vi "Test Xiaolei Hu_Several Frame.vi"() -> ()   [LabVIEW 2017]
doc: "Created IvanLis by LabVIEW Portal\nProfile: http://labviewportal.org/memberlist.php?mode=viewprofile&u=987\neMail: IvanLisanov@gMail.com\nTelegram: https://t.me/IvanLis"
uses:
  libonnx_wrapper/libonnx_wrapper.lvlib
  libonnx_wrapper/TypeDef/IO.ctl
  libonnx_wrapper/TypeDef/Introspection.ctl
panel:
  out "change index":i32
  in  "Next Image":bool
  in  "threshold":sgl=0.3 format="%#.6g"
  in  "max Object's":i64=9
  in  "Tab Control":enum32{"Result", "Introspection"}(tab)
  out "detected_boxes":sgl[][](array[numeric])
  out "detected_classes":sgl[](array[numeric])
  out "score":sgl[](array[numeric])
  out "change":bool[](array[boolean])
  out "Introspection Input":T1
  out "Introspection Output":T1
  out "2D Picture":picture
  out "PNG file path":path=path "/home/ivan/LabVIEWData/ONNX/LabVIEW-ONNX_Runtime/image_for_test/1_1_2r_1_1_var10.jpg"
  out "ONNX model path":path=path "/home/ivan/LabVIEWData/ONNX/LabVIEW-ONNX_Runtime/data/coins_detection.onnx"
  out "error out":errorcluster
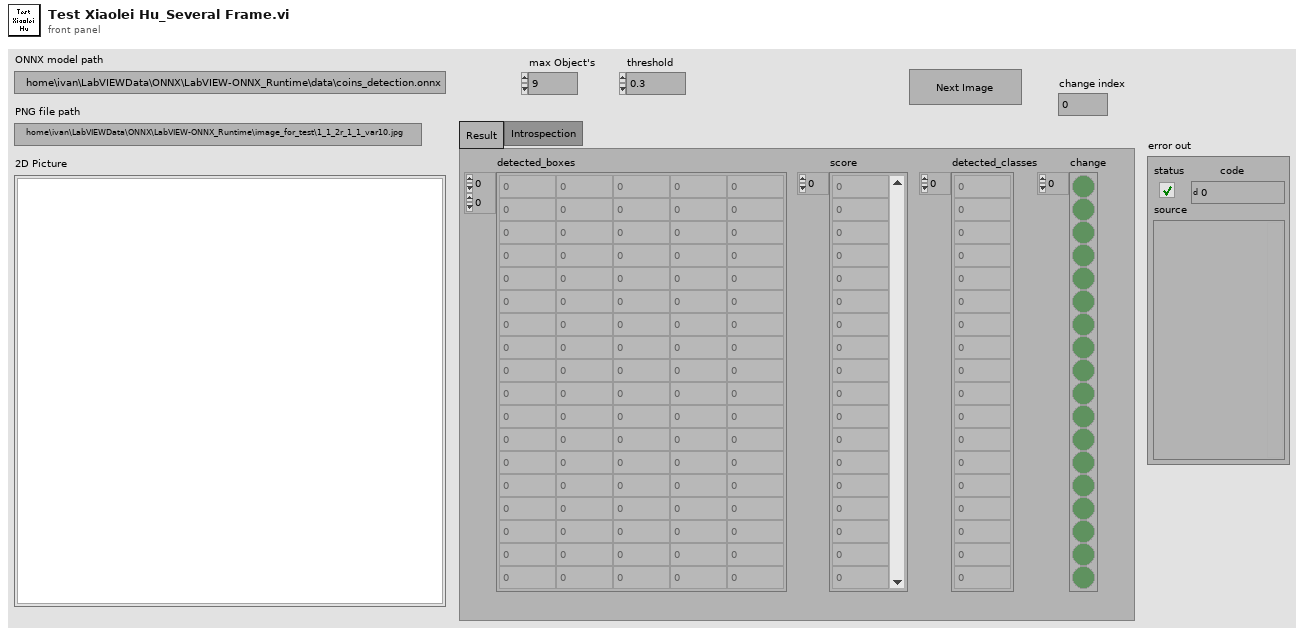
[diagram p1: front panel]
types:
  T1 = typedef "libonnx_wrapper.lvlib/Introspection.ctl" = cluster{"Count":i32, "Shapes":T2[]}
  T2 = typedef "libonnx_wrapper.lvlib/IO.ctl" = cluster{"Name":string, "DimCount":i32, "Type Index":i32, "Type Name":string, "Dims":i64[]}
  T3 = cluster{"left":i16, "top":i16, "right":i16, "bottom":i16}
  T4 = typedef "imagedata.ctl" = cluster{"image type":i32, "image depth":i32, "image":u8[], "mask":u8[], "colors":u32[], "Rectangle":cluster{"left":i16, "top":i16, "right":i16, "bottom":i16}}
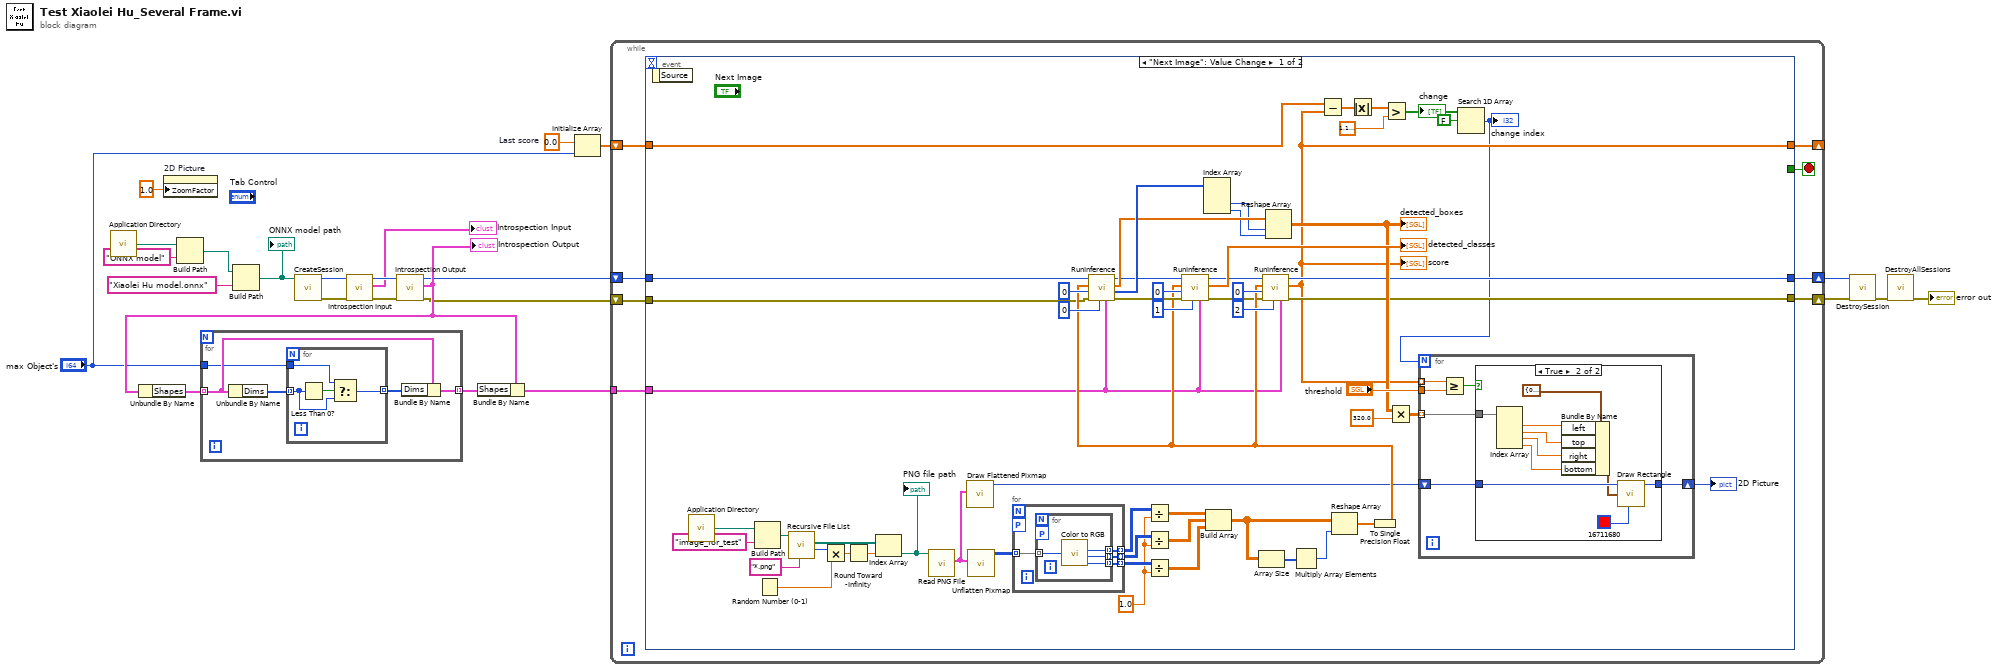
[diagram p0: block diagram]
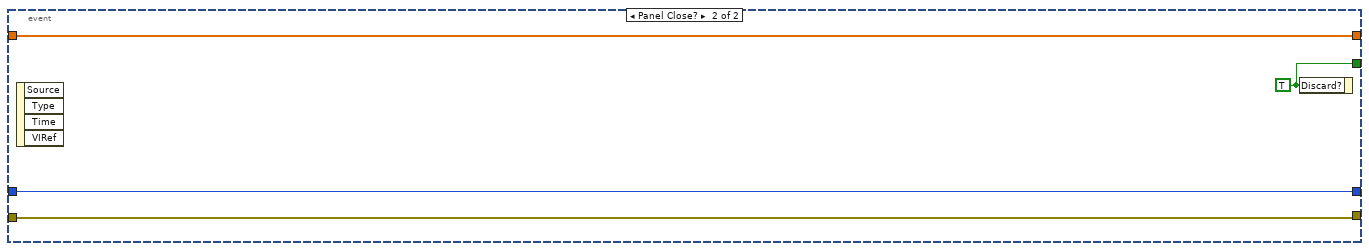
[diagram p3: hidden frame]
diagram:
  w2 = sgl 0.0  # Last score
  n1 = call <vilib>:"Application Directory.vi"() -> ("Application Directory"=w19:path)
  n2 = property on="2D Picture" class="Pict"("ZoomFactor"=sgl 1.0 ("Zoom Factor")) -> ()  [unwired: 2 in, 2 out]
  n3 = Build Path(base path=w19, name or relative path="ONNX model") -> (appended path=w18:path)
  n4 = Build Path(base path=w18, name or relative path="Xiaolei Hu model.onnx") -> (appended path=w20:path)
  "ONNX model path" <- w20
  n5 = call "CreateSession.vi"("ONNX model path"=w20) -> ("error out"=w14:errorcluster, "session id out"=w15:i32)  [unwired: 9 in]
  n6 = call "Introspection Input.vi"("error in (no error)"=w14, "session id in"=w15) -> ("error out"=w16:errorcluster, "Introspection Input"=→"Introspection Input":T1, "session id out"=w17:i32)  [unwired: 7 in]
  n7 = call "Introspection Output.vi"("error in (no error)"=w16, "session id in"=w17) -> ("error out"=w5:errorcluster, "Introspection Output"=w10:T1, "session id out"=w4:i32)  [unwired: 7 in]
  "Introspection Output" <- w10
  n8 = Unbundle By Name(w10) -> ("Shapes"=w12:T2[])
  n9 = for {
    tunnel: w12 -> [w28] mode=indexing
    tunnel: [w26] -> w11 mode=indexing
    tunnel: "max Object's" -> [w25]
    n10 = Unbundle By Name(w28) -> ("Dims"=w29:i64[])
    n11 = for {
      tunnel: w29 -> [w32] mode=indexing
      tunnel: [w31] -> w27 mode=indexing
      tunnel: w25 -> [w30]
      n12 = Less Than 0?(x=w32) -> (x < 0?=w33:bool)
      n13 = Select(t=w30, s=w33, f=w32) -> (s? t:f=w31:i64)
    }
    n14 = Bundle By Name(cluster=w28, "Dims"=w27) -> (w26:T2)
  }
  n15 = Bundle By Name(cluster=w10, "Shapes"=w11) -> (w6:T1)
  n16 = Initialize Array(w2, "max Object's") -> (w3:sgl[])
  n17 = while {
    tunnel: w6 -> [w38]
    shift-right: [w39] -> w21
    shift-left: w4 -> [w36]
    shift-right: [w40] -> w22
    shift-left: w5 -> [w37]
    shift-right: [w34] -> _
    shift-left: w3 -> [w35]
    stop <- w41 stop-if-true
    n18 = event shown="[0] \"Next Image\": Value Change" {
      selector: _ -> [_ _]
      dyn-events: _ -> [_ _]
      timeout: _ -> [_ _]
      tunnel: [_ w128] -> w41
      tunnel: [w54 w126] -> w40
      tunnel: [w53 w127] -> w39
      tunnel: w38 -> [w52 _]
      tunnel: w37 -> [w51 w126]
      tunnel: w36 -> [w50 w127]
      tunnel: w35 -> [w49 w125]
      tunnel: [w48 w125] -> w34
      event "Next Image": Value Change {
        w88 = 1.0 ("y")
        n19 = event-data() -> ()  [unwired: 1 in, 1 out]
        n20 = call <vilib>:"Application Directory.vi"() -> ("Application Directory"=w69:path)
        n21 = Build Path(base path=w69, name or relative path="image_for_test") -> (appended path=w68:path)
        n22 = Random Number (0-1)() -> (number: 0 to 1=w66:dbl)
        n23 = call <vilib>:"Recursive File List.vi"("pattern"="*.png", "Folder Path"=w68) -> ("Number of Files"=w65:i32, "All Files in Dir"=w63:path[])  [unwired: 5 in, 3 out]
        n24 = Multiply(x=w65, y=w66) -> (x*y=w64:dbl)
        n25 = Round Toward -Infinity(1:w64) -> (0:w62:dbl)
        n26 = Index Array(array=w63, index=w62) -> (element=w55:path)
        "PNG file path" <- w55
        n27 = call <vilib>:"Read PNG File.vi"("path to PNG file"=w55) -> ("image data"=w87:T4)  [unwired: 8 in, 2 out]
        n28 = call <vilib>:"Draw Flattened Pixmap.vi"("image data"=w87) -> ("new picture"=w61:picture)  [unwired: 8 in]
        n29 = call <vilib>:"Unflatten Pixmap.vi"("image data"=w87) -> ("24-bit pixmap"=w99:u32[][])  [unwired: 10 out]
        n30 = for {
          tunnel: w99 -> [w120] mode=indexing
          tunnel: [w119] -> w89 mode=indexing
          tunnel: [w118] -> w90 mode=indexing
          tunnel: [w117] -> w91 mode=indexing
          workers-P: _ -> [_]
          n31 = for {
            tunnel: w120 -> [w121] mode=indexing
            tunnel: [w124] -> w119 mode=indexing
            tunnel: [w123] -> w118 mode=indexing
            tunnel: [w122] -> w117 mode=indexing
            workers-P: _ -> [_]
            n32 = call <vilib>:"Color to RGB.vi"("Color"=w121) -> ("R"=w124:u8, "G"=w123:u8, "B"=w122:u8)  [unwired: 1 out]
          }
        }
        n33 = Divide(x=w89, y=w88) -> (x/y=w92:dbl[][])
        n34 = Divide(x=w90, y=w88) -> (x/y=w93:dbl[][])
        n35 = Divide(x=w91, y=w88) -> (x/y=w94:dbl[][])
        n36 = Build Array(w92, w93, w94) -> (w96:dbl[][][])
        n37 = Array Size(array=w96) -> (size(s)=w95:i32[])
        n38 = Multiply Array Elements(1:w95) -> (0:w97:i32)
        n39 = Reshape Array(w96, w97) -> (w98:dbl[])
        n40 = To Single Precision Float(number=w98) -> (single precision float=w72:sgl[])
        n41 = call "RunInference.vi"("Introspection Output"=w52, "outputIndex"=0, "error in (no error)"=w51, "inputIndex"=0, "inputBuffer"=w72, "session id in"=w50) -> ("error out"=w77:errorcluster, "Dims"=w84:i64[], "outputBuffer"=w83:sgl[], "session id out"=w79:i32)  [unwired: 2 in]
        n42 = call "RunInference.vi"("Introspection Output"=w52, "outputIndex"=1, "error in (no error)"=w77, "inputIndex"=0, "inputBuffer"=w72, "session id in"=w79) -> ("error out"=w71:errorcluster, "outputBuffer"=→"detected_classes":sgl[], "session id out"=w73:i32)  [unwired: 2 in, 1 out]
        n43 = Index Array(array=w84) -> (element #2=w82:i64, element #3=w81:i64)  [unwired: 3 in, 1 out]
        n44 = call "RunInference.vi"("Introspection Output"=w52, "outputIndex"=2, "error in (no error)"=w71, "inputIndex"=0, "inputBuffer"=w72, "session id in"=w73) -> ("error out"=w54:errorcluster, "outputBuffer"=w48:sgl[], "session id out"=w53:i32)  [unwired: 2 in, 1 out]
        "score" <- w48
        n45 = Reshape Array(w83, w82, w81) -> (w58:sgl[][])
        "detected_boxes" <- w58
        n46 = Subtract(x=w49, y=w48) -> (x-y=w47:sgl[])
        n47 = Absolute Value(x=w47) -> (abs(x)=w46:sgl[])
        n48 = Greater?(x=w46, y=sgl 1.1920929e-07) -> (0:w44:bool[])
        "change" <- w44
        n49 = Multiply(x=w58, y=sgl 320.0) -> (x*y=w57:sgl[][])
        n50 = Search 1D Array(1D array=w44, element=FALSE) -> (index of element=w42:i32)  [unwired: 1 in]
        "change index" <- w42
        n51 = for {
          N: w42 -> [_]
          tunnel: w48 -> [w105] mode=indexing
          shift-right: [w100] -> w56
          shift-left: w61 -> [w102]
          tunnel: "threshold" -> [w104]
          tunnel: w57 -> [w101] mode=indexing
          n52 = Greater Or Equal?(x=w105, y=w104) -> (x >= y?=w103:bool)
          n53 = case shown="True" w103 {
            tunnel: w102 -> [w106 w116]
            tunnel: w101 -> [_ w115]
            tunnel: [w106 w114] -> w100
            frame False {
            }
            frame True {
              n54 = Index Array(array=w115) -> (element #1=w110:sgl, element #2=w109:sgl, element #3=w108:sgl, element #4=w107:sgl)  [unwired: 4 in]
              n55 = Bundle By Name(cluster=T3 {"left"=0, "top"=0, "right"=0, "bottom"=0} ("rect"), "left"=w110, "top"=w109, "right"=w108, "bottom"=w107) -> (w111:T3)
              n56 = call <vilib>:"Draw Rectangle.vi"("picture"=w116, "rect"=w111, "color(black)"=u32 16711680) -> ("new picture"=w114:picture)  [unwired: 6 in]
            }
          }
        }
        "2D Picture" <- w56
      }
      event Panel Close? {
        w128 = TRUE ("Discard?")
        n57 = event-data() -> ()  [unwired: 1 in, 4 out]
        n58 = event-data("Discard?"=w128) -> ()  [unwired: 1 in, 1 out]
      }
    }
  }
  n59 = call "DestroySession.vi"("error in (no error)"=w22, "session id in"=w21) -> ("error out"=w24:errorcluster)  [unwired: 8 in, 1 out]
  n60 = call "DestroyAllSessions.vi"("error in (no error)"=w24) -> ("error out"=→"error out":errorcluster)  [unwired: 10 in]
